vi "Paths Sub-Parser.vi"(2 "error in (no error)":errorcluster, 3 "Transformation Matrix":T1, 4 "Array of Nodes":string[](array[string])) -> (0 "error out":errorcluster, 1 "paths":T2(array[cluster]))   [LabVIEW 2011]
doc: "This VI parses paths found in an SVG file. It outputs colors, transformation matrices and organized arrays of commands used to specify each particular path."
uses:
  <vilib>/Analysis/Matrix/Datatypes/RealMatrix.ctl
  <vilib>/Analysis/baseanly.llb/Real A x B.vi
  <vilib>/Analysis/NI_AALBase.lvlib
  <vilib>/Analysis/Matrix/NI_Matrix.lvlib
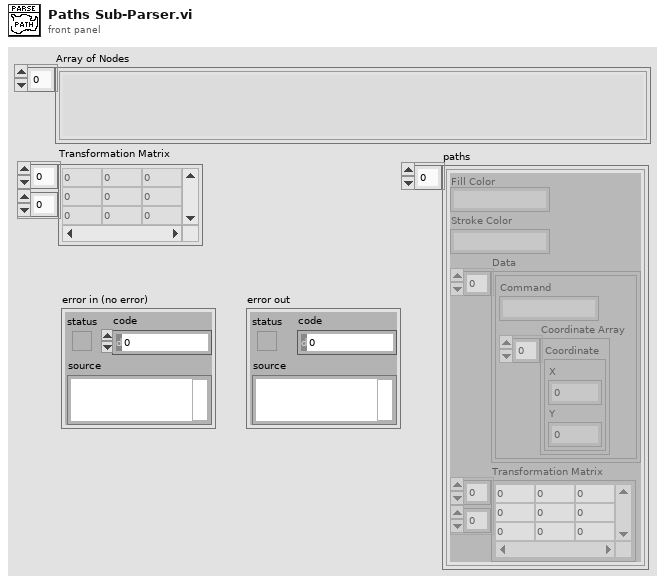
[diagram p1: front panel]
types:
  T1 = typedef "NI_Matrix.lvlib/RealMatrix.ctl" = dbl[][]
  T2 = cluster{"Fill Color":string, "Stroke Color":string, "Data":cluster{"Command":string, "Coordinate Array":cluster{"X":dbl, "Y":dbl}[]}[], "Transformation Matrix":T1}[]
  T3 = cluster{"Command Type":string, "Coordinates":cluster{"X":dbl, "Y":dbl}[]}[]
  T4 = cluster{"XML":string, "XML":string, "Array of Commands":cluster{"Command Type":string, "Coordinates":cluster{"X":dbl, "Y":dbl}[]}[], "Transformation Matrix":T1}
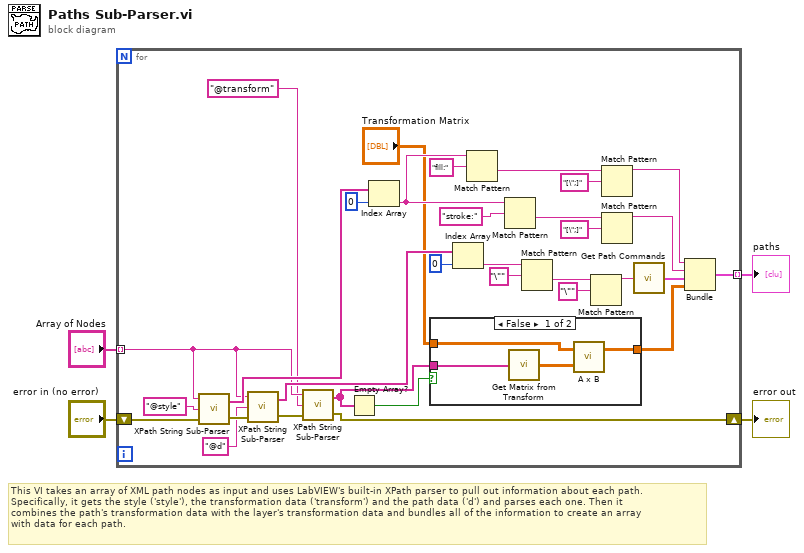
[diagram p0: block diagram]
diagram:
  # "This VI takes an array of XML path nodes as input and uses LabVIEW's built-in XPath parser to pull out information about each path. \nSpecifically, it gets the style ('style'), the transformation data ('transform') and the path data ('d') and parses each one. Then it\ncombines the path's transformation data with the layer's transformation data and bundles all of the information to create an array \nwith data for each path."
  n1 = for {
    tunnel: "Array of Nodes" -> [w10] mode=indexing
    shift-right: [w7] -> w2
    shift-left: "error in (no error)" -> [w30]
    tunnel: [w25] -> w1 mode=indexing
    n2 = call "XPath String Sub-Parser.vi"("error in (no error)"=w30, "XPath expression"="@style", "XML String"=w10) -> ("error out"=w22:errorcluster, "Array of Results"=w35:string[])
    n3 = call "XPath String Sub-Parser.vi"("error in (no error)"=w22, "XPath expression"="@d", "XML String"=w10) -> ("error out"=w8:errorcluster, "Array of Results"=w16:string[])
    n4 = call "XPath String Sub-Parser.vi"("error in (no error)"=w8, "XPath expression"="@transform", "XML String"=w10) -> ("error out"=w7:errorcluster, "Array of Results"=w12:string[])
    n5 = Empty Array?(array=w12) -> (empty?=w11:bool)
    n6 = Index Array(array=w35, index=0) -> (element=w27:string)
    n7 = case shown="False" w11 {
      tunnel: [w40 w41] -> w5
      tunnel: w12 -> [w38 _]
      tunnel: "Transformation Matrix" -> [w37 w41]
      frame False {
        n8 = call "Get Matrix from Transform.vi"("Transform Attributes"=w38) -> ("Matrix"=w39:T1)
        n9 = call-poly <vilib>:"A x B.vi"("B"=w39, "A"=w37) -> ("A x B"=w40:T1)  [unwired: 1 out]
      }
      frame True {
      }
    }
    n10 = Index Array(array=w16, index=0) -> (element=w17:string)
    n11 = Match Pattern(string=w27, regular expression="fill:") -> (after substring=w32:string)  [unwired: 1 in, 3 out]
    n12 = Match Pattern(string=w27, regular expression="stroke:") -> (after substring=w28:string)  [unwired: 1 in, 3 out]
    n13 = Match Pattern(string=w17, regular expression="\"") -> (after substring=w19:string)  [unwired: 1 in, 3 out]
    n14 = Match Pattern(string=w19, regular expression="\"") -> (before substring=w14:string)  [unwired: 1 in, 3 out]
    n15 = Match Pattern(string=w32, regular expression="[\";]") -> (before substring=w24:string)  [unwired: 1 in, 3 out]
    n16 = Match Pattern(string=w28, regular expression="[\";]") -> (before substring=w23:string)  [unwired: 1 in, 3 out]
    n17 = call "Get Path Commands.vi"("Commands Raw Data"=w14) -> ("Array of Commands"=w13:T3)
    n18 = Bundle("XML"=w24, "XML"=w23, "Array of Commands"=w13, "Transformation Matrix"=w5) -> (w25:T4)  [unwired: 1 in]
  }
  "error out" <- w2
  "paths" <- w1
